vi "MQTT_PubAck_Read.vi"(8 "error in (no error)":errorcluster, 11 "connection ID":refnum<k5>) -> (0 "error out":errorcluster, 2 "Message ID":u16=10 format="%x", 3 "connection ID out":refnum<k5>)   [LabVIEW 2012, in "MQTT_Functions.lvlib"]
uses:
  MQTT_Functions.lvlib
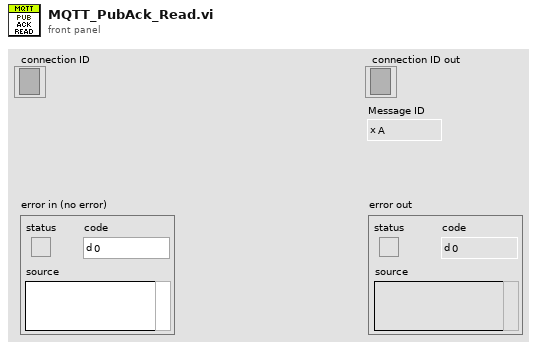
[diagram p1: front panel]
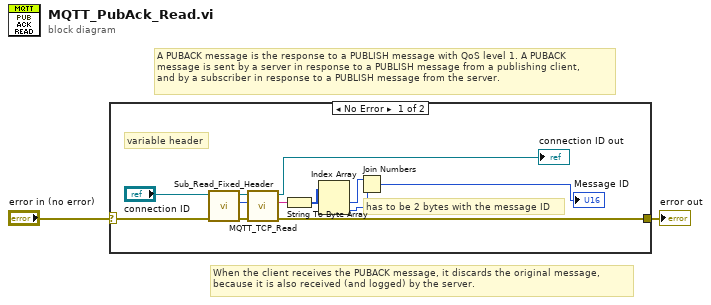
[diagram p0: block diagram]
diagram:
  # "When the client receives the PUBACK message, it discards the original message,\nbecause it is also received (and logged) by the server."
  # "A PUBACK message is the response to a PUBLISH message with QoS level 1. A PUBACK\nmessage is sent by a server in response to a PUBLISH message from a publishing client,\nand by a subscriber in response to a PUBLISH message from the server."
  n1 = case shown="No Error" "error in (no error)" {
    selector: "error in (no error)" -> [w13 w15]
    tunnel: [w6 w15] -> w1
    frame No Error {
      # "has to be 2 bytes with the message ID"
      # "variable header"
      n2 = call "Sub_Read_Fixed_Header.vi"("error in (no error)"=w13, "connection ID"="connection ID") -> ("error out"=w11:errorcluster, "Remaining Length"=w12:u32, "connection ID out"=w10:refnum<k5>)  [unwired: 3 in, 4 out]
      n3 = call "MQTT_TCP_Read.vi"("error in (no error)"=w11, "bytes to read"=w12, "connection ID"=w10) -> ("error out"=w6:errorcluster, "data out"=w9:string, "connection ID out"=→"connection ID out":refnum<k5>)  [unwired: 6 in]
      n4 = String To Byte Array(string=w9) -> (unsigned byte array=w7:u8[])
      n5 = Index Array(array=w7) -> (element #1=w4:u8, element #2=w3:u8)  [unwired: 2 in]
      n6 = Join Numbers(hi=w4, lo=w3) -> ((hi.lo)=→"Message ID":u16)
    }
    frame Error {
    }
  }
  "error out" <- w1
